vi "stress_test_timer.vi"() -> ()   [LabVIEW 2020]
panel:
  in  "Path":path
  out "time for command (ms)":u32
  in  "10000 inserts":string="select * from llab_hello;"
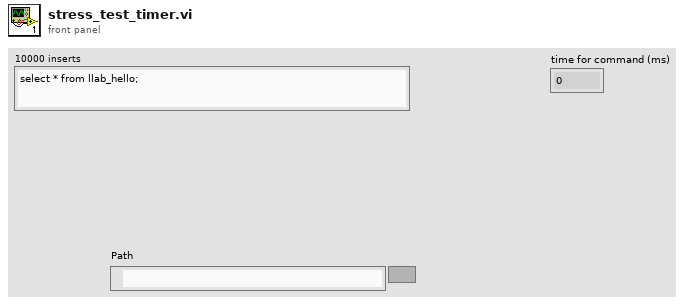
[diagram p1: front panel]
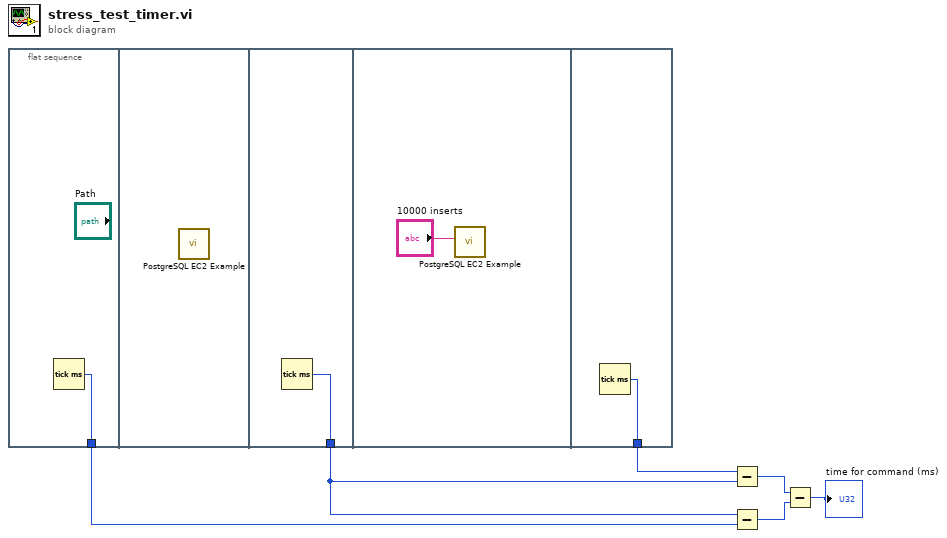
[diagram p0: block diagram]
diagram:
  n1 = flat-sequence {
    tunnel: [w7] -> w6
    tunnel: [w8] -> w5
    tunnel: [w10] -> w2
    frame #0 {
      n2 = Tick Count (ms)() -> (millisecond timer value=w7:u32)
    }
    frame #1 {
      n3 = call "PostgreSQL EC2 Example.vi"() -> ()  [unwired: 11 in, 1 out]
    }
    frame #2 {
      n4 = Tick Count (ms)() -> (millisecond timer value=w8:u32)
    }
    frame #3 {
      n5 = call "PostgreSQL EC2 Example.vi"("command"="10000 inserts") -> ()  [unwired: 10 in, 1 out]
    }
    frame #4 {
      n6 = Tick Count (ms)() -> (millisecond timer value=w10:u32)
    }
  }
  n7 = Subtract(x=w2, y=w5) -> (x-y=w4:u32)
  n8 = Subtract(x=w5, y=w6) -> (x-y=w1:u32)
  n9 = Subtract(x=w4, y=w1) -> (x-y=→"time for command (ms)":u32)
